vi "TI sbRIO Main (FPGA) 9606.vi"() -> ()   [LabVIEW 2013]
uses:
  <vilib>/rvi/Emulation/niFpgaSctlEmulationGetInTimedLoop.vi
  <vilib>/rvi/Emulation/niFpgaEmulationReportErrorSimple.vi
  <vilib>/rvi/Emulation/niFpgaGetClockAttributes.vi
  <vilib>/rvi/eio/common/nirviEmuTemplateMethod_errors.vi
  <vilib>/rvi/Emulation/niFpgaCriticalErrorInLSC.vi
  <vilib>/eio/EIONode/EIONode.xnode
  <vilib>/rvi/FXPMathLib/FxpMul/XNode/nifxpmath_Multiplier.xnode
  <vilib>/rvi/FXPMathLib/sim/FxpSim.dll
  <vilib>/rvi/FXPMathLib/FxpAdd/XNode/nifxpmath_Add.xnode
  <vilib>/Platform/TimedLoop/XDataNode/wakeup.ctl
  <vilib>/Platform/TimedLoop/XDataNode/XDNodeRunTimeDep.lvlib
  <vilib>/Platform/TimedLoop/XDataNode/nitl_modes.ctl
  <vilib>/Platform/TimedLoop/XDataNode/timing_clust.ctl
  <vilib>/Platform/TimedLoop/XDataNode/XDataNode.xnode
  <vilib>/rvi/FXPMathLib/basic elements/FxpIntAccumulator/subVIs/nifxpmath_IntAccumulator_SimConfig.ctl
  <vilib>/rvi/FXPMathLib/basic elements/FxpIntAccumulator/simVIs/DllFxpIntAccumulator_sub.vi
  <vilib>/rvi/FXPMathLib/basic elements/FxpIntAccumulator/XNode/nifxpmath_IntAccumulator.xnode
  <vilib>/fxp/LVFixedPointOverflowPolicyTypeDef.ctl
  <vilib>/rvi/FXPMathLib/FxpSqrt/subVIs/nifxpmath_Sqrt_SimConfig.ctl
  <vilib>/rvi/FXPMathLib/FxpSqrt/simVIs/DllSqrtTemp_sub.vi
  <vilib>/rvi/FXPMathLib/FxpSqrt/XNode/nifxpmath_Sqrt.xnode
  <vilib>/rvi/Analysis/common/codeGenErrors/XNode/niFpgaXNodeCodeGenErrorHandle.vi
  <vilib>/rvi/Analysis/measure/dc-rms/XNode/niFpgaDC-RMS.xnode
  <vilib>/rvi/Analysis/measure/period/templates/niFPGA Period Edge Direction.ctl
  <vilib>/rvi/Analysis/utilities/niFPGA Threshold Crossing Logic.vi
  <vilib>/rvi/Analysis/measure/period/XNode/niFpgaAnalogPeriod.xnode
  <vilib>/rvi/FXPMathLib/FxpDiv/XNode/nifxpmath_Div.xnode
  <vilib>/rvi/Analysis/measure/mean-var-std/XNode/niFpgaMean-Var-Std.xnode
  <vilib>/rvi/FXPMathLib/FxpDiv/simVIs/DllFxpDivTemp_sub.vi
  <vilib>/rvi/FXPMathLib/FxpDiv/subVIs/nifxpmath_Div_SimConfig.ctl
panel:
  out "Elapsed Times":u64[](array[numeric])
  in  "Timer Resets":bool[](array[boolean])=[FALSE, FALSE, FALSE, FALSE, FALSE, FALSE]
  out "Speed (RPM)":fxp<+,32,19>[](array[numeric])
  out "Currents (RMS)":fxp<+,24,6>[](array[numeric]) format="%#.1f"
  in  "Threshold (A)":fxp<+/-,24,6>=1.0
  in  "Consec Samples":i32=125
  out "Actual Pump Starts":u32[](array[numeric])
  in  "Reset":bool
  in  "Duty (Ticks) 6":i32
  in  "Duty (Ticks) 5":i32
  in  "Duty (Ticks) 4":i32
  in  "Duty (Ticks) 3":i32
  in  "PWM Period (Ticks)":u32=40000000
  in  "Duty (Ticks) 1":i32
  in  "Duty (Ticks) 2":i32
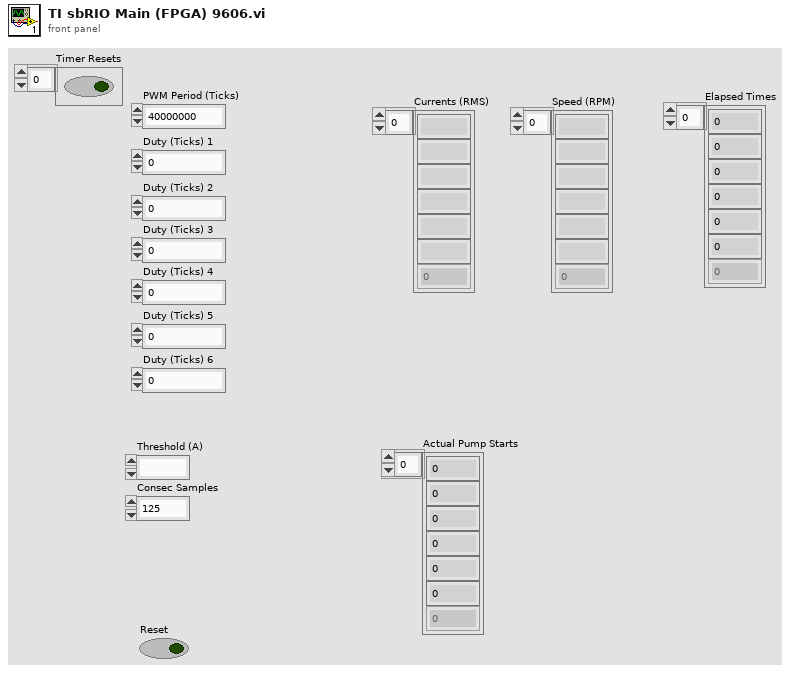
[diagram p1: front panel]
types:
  T1 = typedef "XDNodeRunTimeDep.lvlib/timing_clust.ctl" = cluster{"Expected End [f-1]":u64, "Actual End [f-1]":u64, "Finished Late? [f-1]":bool, "Expected End [i-1]":u64, "Actual End [i-1]":u64, "Finished Late? [i-1]":bool, "Expected Start [i]":u64, "Actual Start [i]":u64, "Expected Start [f]":u64, "Actual Start [f]":u64, "Source Name":string, "Structure Name":string, "Period":i64, "Deadline":i64, "Offset":i64, "Start":i64, "Priority":i32, "Timeout":i32, "Mode":T2, "Wakeup Reason":T3, "Error":errorcluster, "Source Type":string, "Secondary Source Type":string, "Global End Time":u64, "Global Start Time":u64, "Frame Duration":u64, "Iteration Duration":u64, "Assigned CPU":i32, "I/O Scan Engine Mode":u32}
  T2 = typedef "XDNodeRunTimeDep.lvlib/nitl_modes.ctl" = enum32{"No Change", "Process missed periods, maintain original phase", "Discard missed periods, maintain original phase", "Process missed periods, ignore original phase", "Discard missed periods, ignore original phase"}
  T3 = typedef "XDNodeRunTimeDep.lvlib/wakeup.ctl" = enum32{"Normal", "Aborted", "Asynchronous wakeup", "Timing source error", "Timed loop error", "Timeout"}
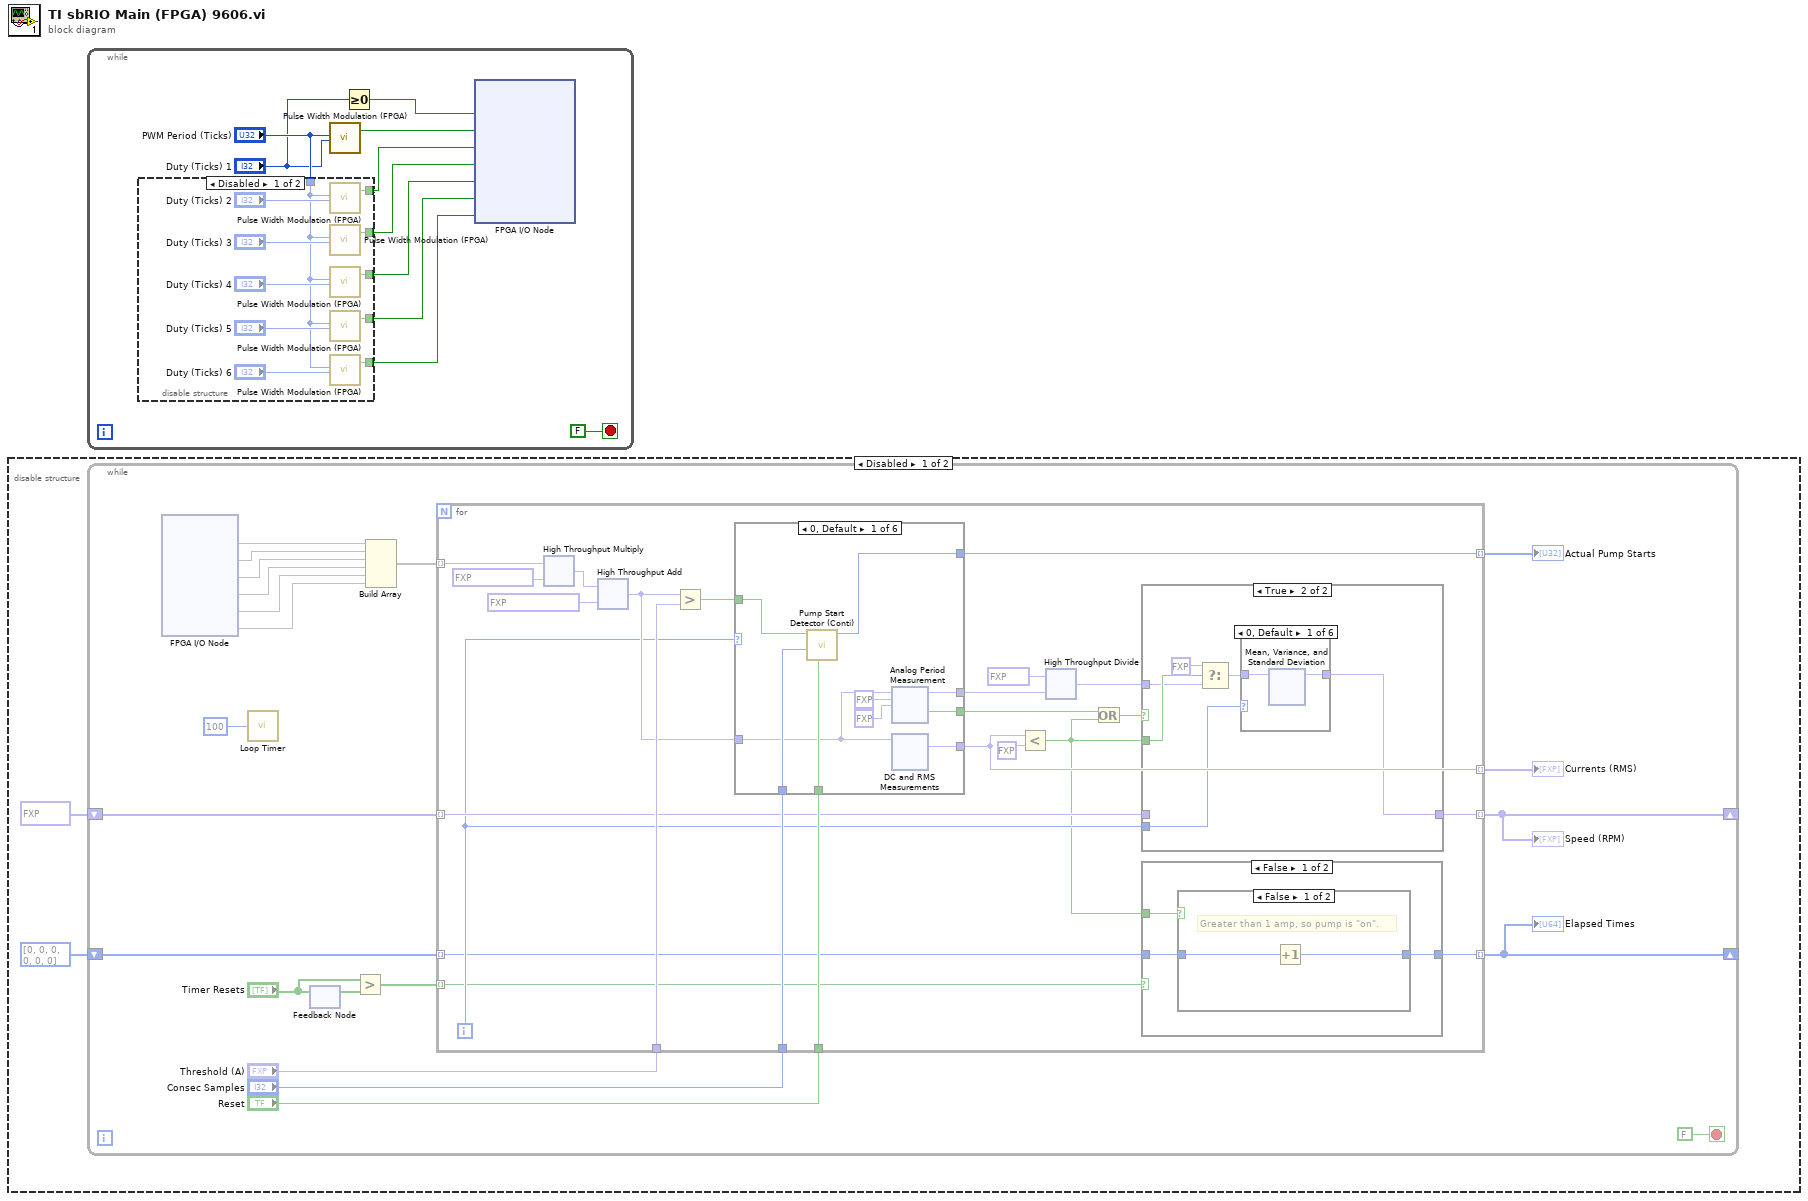
[diagram p0: block diagram]
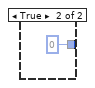
[diagram p3: hidden frame]
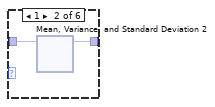
[diagram p5: hidden frame]
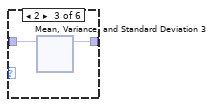
[diagram p6: hidden frame]
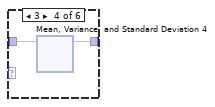
[diagram p7: hidden frame]
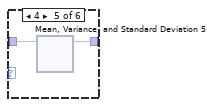
[diagram p8: hidden frame]
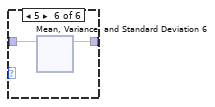
[diagram p9: hidden frame]
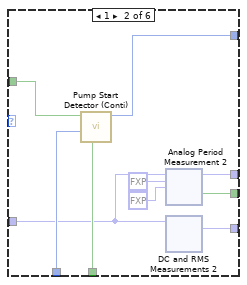
[diagram p10: hidden frame]
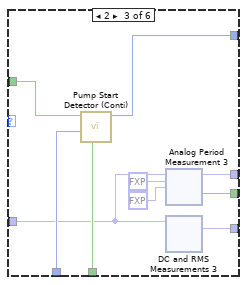
[diagram p11: hidden frame]
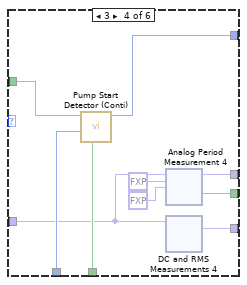
[diagram p12: hidden frame]
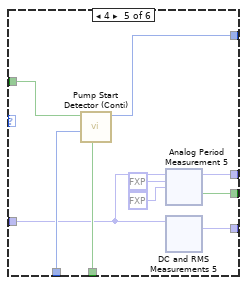
[diagram p13: hidden frame]
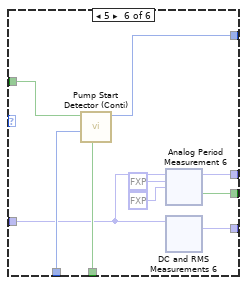
[diagram p14: hidden frame]
diagram:
  n1 = disable-structure shown="Disabled" {
    frame Disabled {
      n2 = while {
        shift-right: [w8] -> _
        shift-left: fxp<+,32,19>[] [0.0, 0.0, 0.0, 0.0, 0.0, 0.0] -> [w9]
        shift-right: [w6] -> _
        shift-left: u64[] [0, 0, 0, 0, 0, 0] -> [w7]
        stop <- FALSE stop-if-true
        n3 = xnode "FPGA I/O Node"() -> ("AI0"=w14, "AI1"=w23, "AI2"=w22, "AI3"=w21, "AI4"=w20, "AI5"=w19)  [unwired: 6 in, 6 out]
        n4 = call "Loop Timer"("Count(uSec)"=u32 100 ("Loop Timer (uSec)")) -> ()  [unwired: 1 out]
        n5 = feedback-in #1("Timer Resets") -> ()
        n6 = feedback #1() -> (w4:bool[])  [unwired: 1 in]
        n7 = Greater?(x="Timer Resets", y=w4) -> (0:w3:bool[])
        n8 = Build Array(w14, w23, w22, w21, w20, w19) -> (w11:void[])
        n9 = for {
          tunnel: "Consec Samples" -> [w47]
          tunnel: [w46] -> w16 mode=indexing
          tunnel: "Threshold (A)" -> [w45]
          tunnel: "Reset" -> [w43]
          tunnel: w11 -> [w39] mode=indexing
          tunnel: [w35] -> w10 mode=indexing
          tunnel: w7 -> [w26] mode=indexing
          tunnel: [w25] -> w6 mode=indexing
          tunnel: w9 -> [w31] mode=indexing
          tunnel: [w30] -> w8 mode=indexing
          tunnel: w3 -> [w24] mode=indexing
          i -> [w29]
          n10 = xnode ("High Throughput Multiply")("x"=w39, "y"=fxp<+,16,5> 24.0380859375) -> ("x*y"=w41:fxp<+/-,40,10>)
          n11 = xnode ("High Throughput Add")("x"=w41, "y"=fxp<+/-,18,7> -60.09521484375) -> ("x+y"=w38:fxp<+/-,24,6>)
          n12 = Greater?(x=w38, y=w45) -> (0:w44:bool)
          n13 = case shown="0, Default" w29 {
            tunnel: w44 -> [w566 w799 w1032 w1265 w1498 w1731]
            tunnel: w47 -> [w565 w798 w1031 w1264 w1497 w1730]
            tunnel: [w564 w797 w1030 w1263 w1496 w1729] -> w46
            tunnel: w43 -> [w563 w796 w1029 w1262 w1495 w1728]
            tunnel: w38 -> [w560 w793 w1026 w1259 w1492 w1725]
            tunnel: [w559 w792 w1025 w1258 w1491 w1724] -> w35
            tunnel: [w558 w791 w1024 w1257 w1490 w1723] -> w32
            tunnel: [w557 w790 w1023 w1256 w1489 w1722] -> w28
            frame 0, Default {
              n14 = call "Pump Start Detector (Conti).vi"("Reset"=w563, "Consec Samples"=w565, "Crossing?"=w566) -> ("Restarts"=w564:u32)  [unwired: 8 in]
              n15 = xnode ("Analog Period Measurement")("input data"=w560, "threshold level"=fxp<+/-,24,6> 0.0, "hysteresis"=fxp<+,23,5> 1.0) -> ("period (samples)"=w557:fxp<+,32,16>, "output valid"=w558:bool)  [unwired: 2 in, 2 out]
              n16 = xnode ("DC and RMS Measurements")("input data"=w560) -> ("RMS"=w559:fxp<+,24,6>)  [unwired: 1 in, 1 out]
            }
            frame 1 {
              n17 = call "Pump Start Detector (Conti).vi"("Reset"=w796, "Consec Samples"=w798, "Crossing?"=w799) -> ("Restarts"=w797:u32)  [unwired: 8 in]
              n18 = xnode ("Analog Period Measurement 2")("input data"=w793, "threshold level"=fxp<+/-,24,6> 0.0, "hysteresis"=fxp<+,23,5> 1.0) -> ("period (samples)"=w790:fxp<+,32,16>, "output valid"=w791:bool)  [unwired: 2 in, 2 out]
              n19 = xnode ("DC and RMS Measurements 2")("input data"=w793) -> ("RMS"=w792:fxp<+,24,6>)  [unwired: 1 in, 1 out]
            }
            frame 2 {
              n20 = call "Pump Start Detector (Conti).vi"("Reset"=w1029, "Consec Samples"=w1031, "Crossing?"=w1032) -> ("Restarts"=w1030:u32)  [unwired: 8 in]
              n21 = xnode ("Analog Period Measurement 3")("input data"=w1026, "threshold level"=fxp<+/-,24,6> 0.0, "hysteresis"=fxp<+,23,5> 1.0) -> ("period (samples)"=w1023:fxp<+,32,16>, "output valid"=w1024:bool)  [unwired: 2 in, 2 out]
              n22 = xnode ("DC and RMS Measurements 3")("input data"=w1026) -> ("RMS"=w1025:fxp<+,24,6>)  [unwired: 1 in, 1 out]
            }
            frame 3 {
              n23 = call "Pump Start Detector (Conti).vi"("Reset"=w1262, "Consec Samples"=w1264, "Crossing?"=w1265) -> ("Restarts"=w1263:u32)  [unwired: 8 in]
              n24 = xnode ("Analog Period Measurement 4")("input data"=w1259, "threshold level"=fxp<+/-,24,6> 0.0, "hysteresis"=fxp<+,23,5> 1.0) -> ("period (samples)"=w1256:fxp<+,32,16>, "output valid"=w1257:bool)  [unwired: 2 in, 2 out]
              n25 = xnode ("DC and RMS Measurements 4")("input data"=w1259) -> ("RMS"=w1258:fxp<+,24,6>)  [unwired: 1 in, 1 out]
            }
            frame 4 {
              n26 = call "Pump Start Detector (Conti).vi"("Reset"=w1495, "Consec Samples"=w1497, "Crossing?"=w1498) -> ("Restarts"=w1496:u32)  [unwired: 8 in]
              n27 = xnode ("Analog Period Measurement 5")("input data"=w1492, "threshold level"=fxp<+/-,24,6> 0.0, "hysteresis"=fxp<+,23,5> 1.0) -> ("period (samples)"=w1489:fxp<+,32,16>, "output valid"=w1490:bool)  [unwired: 2 in, 2 out]
              n28 = xnode ("DC and RMS Measurements 5")("input data"=w1492) -> ("RMS"=w1491:fxp<+,24,6>)  [unwired: 1 in, 1 out]
            }
            frame 5 {
              n29 = call "Pump Start Detector (Conti).vi"("Reset"=w1728, "Consec Samples"=w1730, "Crossing?"=w1731) -> ("Restarts"=w1729:u32)  [unwired: 8 in]
              n30 = xnode ("Analog Period Measurement 6")("input data"=w1725, "threshold level"=fxp<+/-,24,6> 0.0, "hysteresis"=fxp<+,23,5> 1.0) -> ("period (samples)"=w1722:fxp<+,32,16>, "output valid"=w1723:bool)  [unwired: 2 in, 2 out]
              n31 = xnode ("DC and RMS Measurements 6")("input data"=w1725) -> ("RMS"=w1724:fxp<+,24,6>)  [unwired: 1 in, 1 out]
            }
          }
          n32 = Less?(x=w35, y=fxp<+,24,6> 1.0 ("current threshold")) -> (x < y?=w27:bool)
          n33 = xnode "High Throughput Divide"("x"=fxp<+,32,19> 300000.0, "y"=w28) -> ("x/y"=w33:fxp<+,32,18>)
          n34 = Or(x=w32, y=w27) -> (x .or. y?=w34:bool)
          n35 = case shown="True" w34 {
            tunnel: w33 -> [_ w59]
            tunnel: w27 -> [_ w60]
            tunnel: w31 -> [w55 _]
            tunnel: [w55 w56] -> w30
            tunnel: w29 -> [_ w58]
            frame False {
            }
            frame True {
              n36 = Select(t=fxp<+,32,18> 0.0 ("input data"), s=w60, f=w59) -> (s? t:f=w57:fxp<+,32,18>)
              n37 = case shown="0, Default" w58 {
                tunnel: w57 -> [w63 w141 w219 w297 w375 w453]
                tunnel: [w62 w140 w218 w296 w374 w452] -> w56
                frame 0, Default {
                  n38 = xnode ("Mean, Variance, and Standard Deviation")("input data"=w63) -> ("mean"=w62:fxp<+/-,32,19>)  [unwired: 1 in, 1 out]
                }
                frame 1 {
                  n39 = xnode ("Mean, Variance, and Standard Deviation 2")("input data"=w141) -> ("mean"=w140:fxp<+/-,32,19>)  [unwired: 1 in, 1 out]
                }
                frame 2 {
                  n40 = xnode ("Mean, Variance, and Standard Deviation 3")("input data"=w219) -> ("mean"=w218:fxp<+/-,32,19>)  [unwired: 1 in, 1 out]
                }
                frame 3 {
                  n41 = xnode ("Mean, Variance, and Standard Deviation 4")("input data"=w297) -> ("mean"=w296:fxp<+/-,32,19>)  [unwired: 1 in, 1 out]
                }
                frame 4 {
                  n42 = xnode ("Mean, Variance, and Standard Deviation 5")("input data"=w375) -> ("mean"=w374:fxp<+/-,32,19>)  [unwired: 1 in, 1 out]
                }
                frame 5 {
                  n43 = xnode ("Mean, Variance, and Standard Deviation 6")("input data"=w453) -> ("mean"=w452:fxp<+/-,32,19>)  [unwired: 1 in, 1 out]
                }
              }
            }
          }
          n44 = case shown="False" w24 {
            tunnel: w27 -> [w50 _]
            tunnel: w26 -> [w49 _]
            tunnel: [w48 u64 0] -> w25
            frame False {
              n45 = case shown="False" w50 {
                tunnel: w49 -> [w52 w53]
                tunnel: [w51 w53] -> w48
                frame False {
                  # "Greater than 1 amp, so pump is \"on\"."
                  n46 = Increment(x=w52) -> (x+1=w51:u64)
                }
                frame True {
                }
              }
            }
            frame True {
            }
          }
        }
        "Actual Pump Starts" <- w16
        "Currents (RMS)" <- w10
        "Speed (RPM)" <- w8
        "Elapsed Times" <- w6
      }
    }
    frame Enabled {
    }
  }
  n47 = while {
    stop <- FALSE stop-if-true
    n48 = disable-structure shown="Disabled" {
      disable-tunnel: [w1974 _] -> w1963
      disable-tunnel: "PWM Period (Ticks)" -> [w1969 _]
      disable-tunnel: [w1968 _] -> w1961
      disable-tunnel: [w1967 _] -> w1960
      disable-tunnel: [w1966 _] -> w1959
      disable-tunnel: [w1965 _] -> w1958
      frame Disabled {
        n49 = call "Pulse Width Modulation (FPGA).vi"("PWM Period (Ticks)"=w1969, "PWM Duty Cycle (Ticks)"="Duty (Ticks) 2") -> ("PWM DO"=w1974:bool)  [unwired: 14 in, 3 out]
        n50 = call "Pulse Width Modulation (FPGA).vi"("PWM Period (Ticks)"=w1969, "PWM Duty Cycle (Ticks)"="Duty (Ticks) 3") -> ("PWM DO"=w1968:bool)  [unwired: 14 in, 3 out]
        n51 = call "Pulse Width Modulation (FPGA).vi"("PWM Period (Ticks)"=w1969, "PWM Duty Cycle (Ticks)"="Duty (Ticks) 4") -> ("PWM DO"=w1967:bool)  [unwired: 14 in, 3 out]
        n52 = call "Pulse Width Modulation (FPGA).vi"("PWM Period (Ticks)"=w1969, "PWM Duty Cycle (Ticks)"="Duty (Ticks) 5") -> ("PWM DO"=w1966:bool)  [unwired: 14 in, 3 out]
        n53 = call "Pulse Width Modulation (FPGA).vi"("PWM Period (Ticks)"=w1969, "PWM Duty Cycle (Ticks)"="Duty (Ticks) 6") -> ("PWM DO"=w1965:bool)  [unwired: 14 in, 3 out]
      }
      frame Enabled {
      }
    }
    n54 = call "Pulse Width Modulation (FPGA).vi"("PWM Period (Ticks)"="PWM Period (Ticks)", "PWM Duty Cycle (Ticks)"="Duty (Ticks) 1") -> ("PWM DO"=w1964:bool)  [unwired: 14 in, 3 out]
    n55 = Greater Or Equal To 0?(x="Duty (Ticks) 1") -> (x >= 0?=w1955:bool)
    n56 = xnode "FPGA I/O Node"("RMC/DIO6"=w1955, "RMC/DIO0"=w1964, "RMC/DIO1"=w1963, "RMC/DIO2"=w1961, "RMC/DIO3"=w1960, "RMC/DIO4"=w1959, "RMC/DIO5"=w1958) -> ()  [unwired: 8 in, 8 out]
  }
